vi "Segment_c.vi"(11 "Input in Binary":bool[](array[boolean])) -> (3 "Segment c":bool)   [LabVIEW 2024]
panel:
  out "D":bool
  out "C":bool
  out "B":bool
  out "A":bool
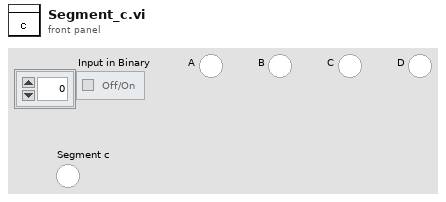
[diagram p1: front panel]
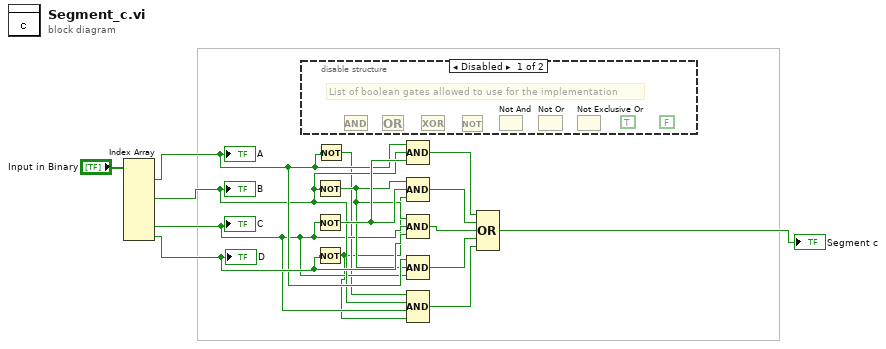
[diagram p0: block diagram]
diagram:
  n1 = Index Array(array="Input in Binary") -> (element #5=w12:bool, element #6=w10:bool, element #7=w9:bool, element #8=w13:bool)  [unwired: 8 in, 4 out]
  "A" <- w12
  "B" <- w10
  "C" <- w9
  "D" <- w13
  n2 = disable-structure shown="Disabled" {
    frame Disabled {
      (unwired) FALSE
      (unwired) TRUE
      # "List of boolean gates allowed to use for the implementation"
      n3 = And() -> ()  [unwired: 2 in, 1 out]
      n4 = Or() -> ()  [unwired: 2 in, 1 out]
      n5 = Exclusive Or() -> ()  [unwired: 2 in, 1 out]
      n6 = Not() -> ()  [unwired: 1 in, 1 out]
      n7 = Not And() -> ()  [unwired: 2 in, 1 out]
      n8 = Not Or() -> ()  [unwired: 2 in, 1 out]
      n9 = Not Exclusive Or() -> ()  [unwired: 2 in, 1 out]
    }
    frame Enabled {
    }
  }
  n10 = Not(x=w10) -> (.not. x?=w11:bool)
  n11 = Not(x=w9) -> (.not. x?=w14:bool)
  n12 = Not(x=w13) -> (.not. x?=w7:bool)
  n13 = Not(x=w12) -> (.not. x?=w8:bool)
  n14 = Compound Arithmetic op=AND(w12, w10, w14) -> (w5:bool)
  n15 = Compound Arithmetic op=AND(w11, w14, w7) -> (w4:bool)
  n16 = Compound Arithmetic op=AND(w11, w9, w13) -> (w3:bool)
  n17 = Compound Arithmetic op=AND(w12, w11, w9) -> (w2:bool)
  n18 = Compound Arithmetic op=AND(w8, w10, w9, w7) -> (w1:bool)
  n19 = Compound Arithmetic op=OR(w5, w4, w3, w2, w1) -> (→"Segment c":bool)
